vi "Load from Folder (Factory).vi"(7 "Logger":refnum<class "Logger.lvclass">, 8 "error in (no error)":errorcluster, 10 "Folder":path) -> (0 "error out":errorcluster, 3 "PackageAbstract out":refnum<class "PackageAbstract.lvclass">)   [LabVIEW 2020, in "GPack.lvlib" / "PackageAbstract.lvclass"]
uses:
  PackageAbstract.lvclass
  C:/dev/lv20CE/lv-gpack/GPack/Package/Package.lvclass
  Logger/Logger.lvclass
  GPack File/GPack File.lvclass
  PackageAbstract.lvclass/PackageAbstract.ctl
  GPack.lvlib
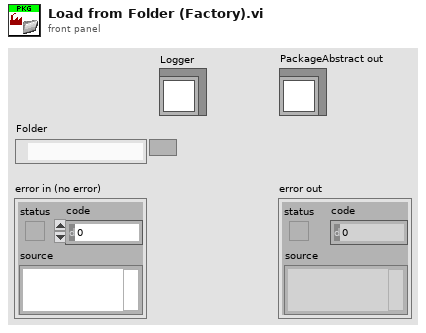
[diagram p1: front panel]
types:
  T1 = typedef "GPack.lvlib/Dependency.ctl" = cluster{"Info":T2, "Path":path}
  T2 = typedef "GPack.lvlib/Package Info.ctl" = cluster{"Name":string, "Type":string, "Host":string, "Path":string, "Branch":string, "Version":string, "License":string}
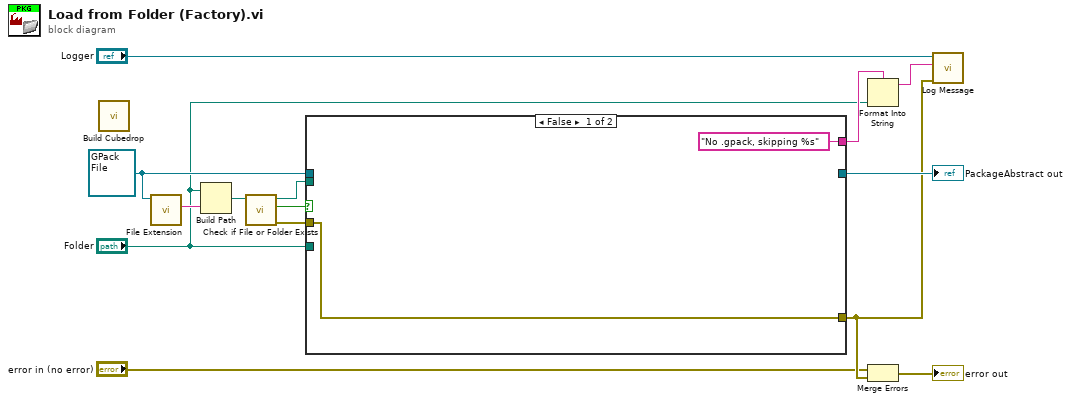
[diagram p0: block diagram]
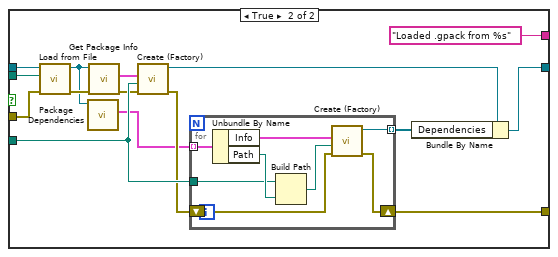
[diagram p2: hidden frame]
diagram:
  w12 = refnum<class "GPack File.lvclass"> refnum ("GPack File in")
  n1 = call "Build Cubedrop.vi"() -> ()  [unwired: 12 in]
  n2 = call-dynamic "File Extension.vi"("GPack File in"=w12) -> ("File Extension"=w13:string)  [unwired: 9 in, 1 out]
  n3 = Build Path(base path="Folder", name or relative path=w13) -> (appended path=w9:path)
  n4 = call <vilib>:"Check if File or Folder Exists.vi"("path"=w9) -> ("error out"=w7:errorcluster, "file or folder exists?"=w8:bool, "dup path"=w6:path)  [unwired: 8 in]
  n5 = case shown="False" w8 {
    tunnel: [w15 w30] -> w3
    tunnel: [_ w29] -> w14
    tunnel: "Folder" -> [_ w28]
    tunnel: w12 -> [_ w25]
    tunnel: w7 -> [w15 w19]
    tunnel: w6 -> [_ w18]
    tunnel: ["No .gpack, skipping %s" ("format string") "Loaded .gpack from %s" ("format string")] -> w5
    frame False {
    }
    frame True {
      n6 = call-dynamic "Load from File.vi"("error in (no error)"=w19, "Path"=w18, "GPack File in"=w25) -> ("error out"=w26:errorcluster, "GPack File out"=w23:refnum<class "GPack File.lvclass">)  [unwired: 7 in]
      n7 = call-dynamic "Package Dependencies.vi"("GPack File in"=w23) -> ("Dependencies"=w22:T1[])  [unwired: 9 in, 1 out]
      n8 = call "Get Package Info.vi"("GPack File in"=w23) -> ("Package Info"=w24:T2)  [unwired: 10 in]
      n9 = call "Create (Factory).vi"("error in (no error)"=w26, "Folder"=w28, "Package Info"=w24) -> ("error out"=w27:errorcluster, "PackageAbstract out"=w21:refnum<class "PackageAbstract.lvclass">)  [unwired: 7 in]
      n10 = for {
        tunnel: w22 -> [w38] mode=indexing
        shift-right: [w35] -> w30
        shift-left: w27 -> [w36]
        tunnel: [w34] -> w20 mode=indexing
        tunnel: w28 -> [w31]
        n11 = Unbundle By Name(w38) -> ("Info"=w37:T2, "Path"=w33:path)
        n12 = Build Path(base path=w31, name or relative path=w33) -> (appended path=w32:path)
        n13 = call "Create (Factory).vi"("error in (no error)"=w36, "Folder"=w32, "Package Info"=w37) -> ("error out"=w35:errorcluster, "PackageAbstract out"=w34:refnum<class "PackageAbstract.lvclass">)  [unwired: 7 in]
      }
      n14 = Bundle By Name(cluster=w21, "Dependencies"=w20) -> (w29:refnum<class "PackageAbstract.lvclass">)
    }
  }
  "PackageAbstract out" <- w14
  n15 = Format Into String(format string=w5, "Folder") -> (resulting string=w10:string)  [unwired: 2 in, 1 out]
  n16 = Merge Errors("error in (no error)", w3) -> (→"error out":errorcluster)
  n17 = call "Log Message.vi"("error in (no error)"=w3, "Message"=w10, "Logger in"="Logger") -> ()  [unwired: 7 in, 2 out]
